vi "Convert 2D Array to Cluster.vi"(8 "error in (no error)":errorcluster, 11 "Array in":string[][](array[string])) -> (0 "error out":errorcluster, 3 "Array out":T1[](array[typedef]))   [LabVIEW 2025, in "Project.lvclass"]
doc: "Convert 2D Array of strings to Sorted, Structured Cluster of:\n\nFPGA Targets\n-Owned Modules\n--Owned Signals"
uses:
  Project.lvclass
  FPGA Settings.ctl
  Module/Module/Module Settings.ctl
  Signal/Signal/Signal Settings.ctl
  Project.lvclass/Project.ctl
  Signal/Signal/Signal.lvclass
  Module/Module/Module.lvclass
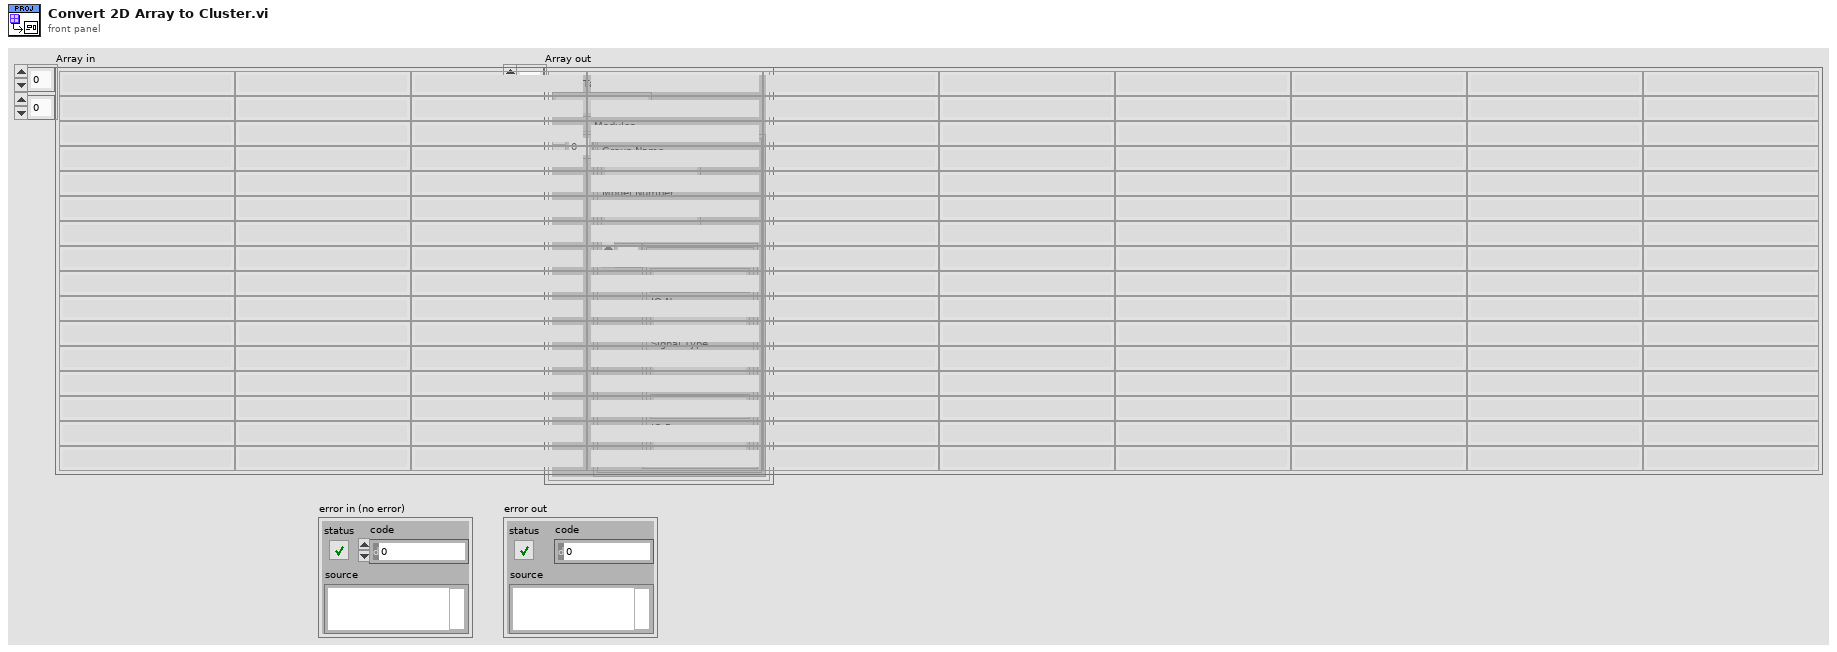
[diagram p1: front panel]
types:
  T1 = typedef "Project.lvclass/FPGA Settings.ctl" = cluster{"FPGA Target Name":string, "Modules":T2[]}
  T2 = typedef "Module.lvclass/Module Settings.ctl" = cluster{"Group Name":string, "Model Number":string, "Signals":T3[]}
  T3 = typedef "Signal.lvclass/Signal Settings.ctl" = cluster{"Signal Name":string, "IO Name":string, "Signal Type":string, "Signal Parameters":string, "IO Resource":string}
  T4 = cluster{"Group Name":string, "Model Number":string, "Signal LUT":variant}
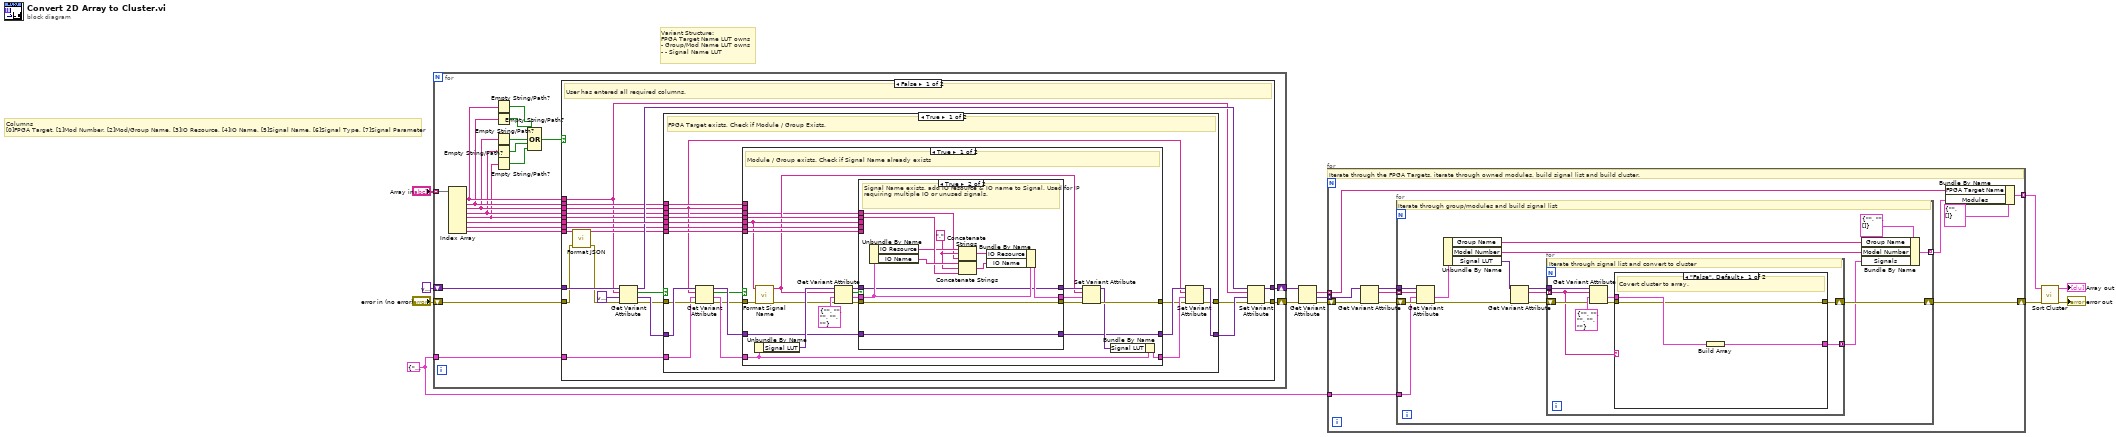
[diagram p0: block diagram]
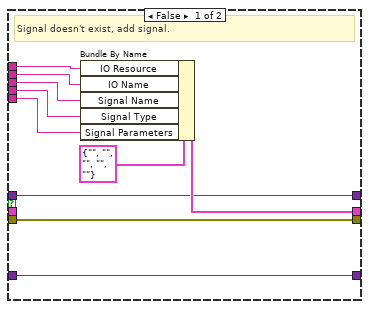
[diagram p2: hidden frame]
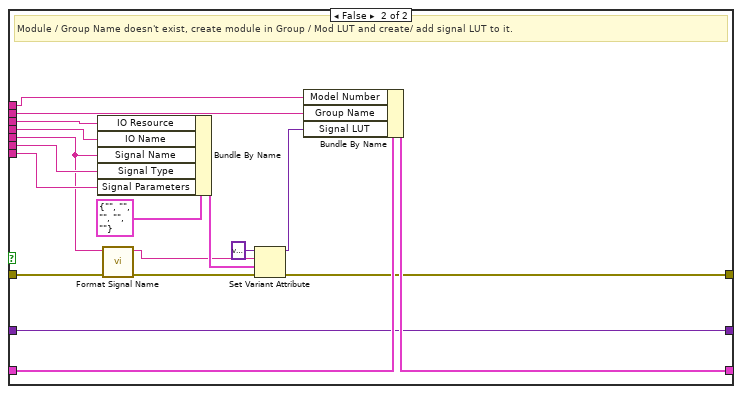
[diagram p3: hidden frame]
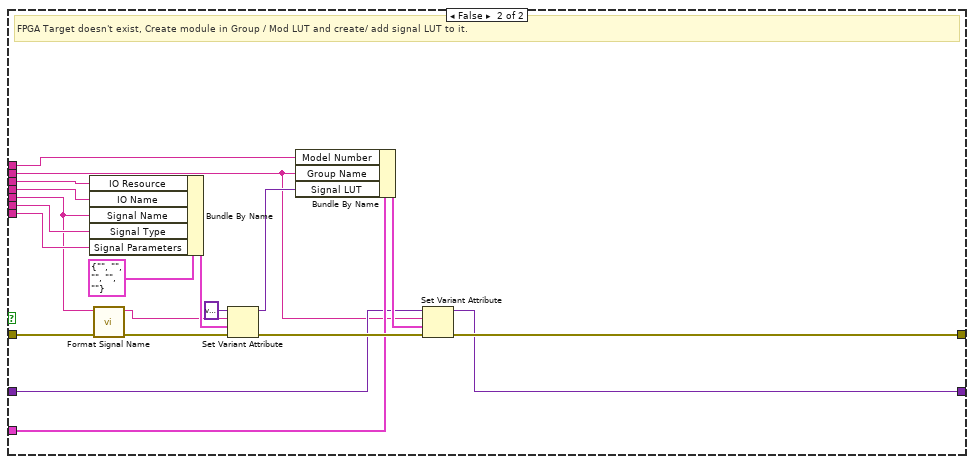
[diagram p4: hidden frame]
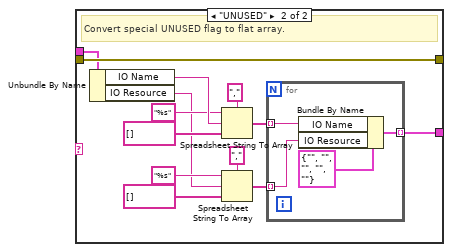
[diagram p6: hidden frame]
diagram:
  w13 = T4 {"Group Name"="", "Model Number"="", "Signal LUT"=variant}
  # "Variant Structure:\nFPGA Target Name LUT owns\n- Group/Mod Name LUT owns\n- - Signal Name LUT"
  # "Columns\n[0]FPGA Target, [1]Mod Number, [2]Mod/Group Name, [3]IO Resource, [4]IO Name, [5]Signal Name, [6]Signal Type, [7]Signal Parameter"
  n1 = for {
    tunnel: "Array in" -> [w32] mode=indexing
    shift-right: [w30] -> w8
    shift-left: variant -> [w33]
    shift-right: [w29] -> w9
    shift-left: "error in (no error)" -> [w28]
    tunnel: w13 -> [w27]
    n2 = Index Array(array=w32) -> (element #1=w24:string, element #2=w23:string, element #3=w22:string, element #4=w21:string, element #5=w20:string, element #6=w31:string, element #7=w25:string, element #8=w26:string)  [unwired: 8 in]
    n3 = Empty String/Path?(string/path=w24) -> (empty?=w19:bool)
    n4 = Empty String/Path?(string/path=w23) -> (empty?=w18:bool)
    n5 = Empty String/Path?(string/path=w22) -> (empty?=w17:bool)
    n6 = Empty String/Path?(string/path=w21) -> (empty?=w16:bool)
    n7 = Empty String/Path?(string/path=w20) -> (empty?=w15:bool)
    n8 = Compound Arithmetic op=OR(w19, w18, w17, w16, w15) -> (w14:bool)
    n9 = case shown="False" w14 {
      tunnel: w33 -> [w55 w158]
      tunnel: w31 -> [w51 _]
      tunnel: [w49 w158] -> w30
      tunnel: [w47 w159] -> w29
      tunnel: w28 -> [w43 w159]
      tunnel: w27 -> [w41 _]
      tunnel: w26 -> [w40 _]
      tunnel: w25 -> [w39 _]
      tunnel: w24 -> [w34 _]
      tunnel: w23 -> [w38 _]
      tunnel: w22 -> [w37 _]
      tunnel: w21 -> [w36 _]
      tunnel: w20 -> [w35 _]
      frame False {
        # "User has entered all required columns."
        n10 = call "Format JSON.vi"("error in (no error)"=w43, "String"=w40) -> ("error out"=w42:errorcluster, "String out"=w44:string)  [unwired: 8 in]
        n11 = Get Variant Attribute(Variant=w55, name=w34, default value (empty Variant)=variant ("default value (empty variant)"), error in=w42) -> (duplicate Variant=w45:variant, found=w54:bool, value=w52:variant, error out=w46:errorcluster)
        n12 = case shown="True" w54 {
          tunnel: w52 -> [w74 w142]
          tunnel: w36 -> [w56 w138]
          tunnel: w35 -> [w59 w147]
          tunnel: w51 -> [w60 w146]
          tunnel: w44 -> [w73 w157]
          tunnel: w37 -> [w57 w139]
          tunnel: w38 -> [w58 w140]
          tunnel: [w65 w141] -> w50
          tunnel: [w64 w155] -> w48
          tunnel: w46 -> [w63 w144]
          tunnel: w41 -> [w62 w149]
          tunnel: w39 -> [w61 w148]
          frame True {
            # "FPGA Target exists, Check if Module / Group Exists."
            n13 = Get Variant Attribute(Variant=w74, name=w57, default value (empty Variant)=w62, error in=w63) -> (duplicate Variant=w70:variant, found=w68:bool, value=w72:T4, error out=w67:errorcluster)
            n14 = case shown="True" w68 {
              tunnel: w59 -> [w97 w136]
              tunnel: w60 -> [w79 w125]
              tunnel: w61 -> [w96 w135]
              tunnel: w73 -> [w95 w134]
              tunnel: w72 -> [w83 w133]
              tunnel: [w80 w123] -> w71
              tunnel: w70 -> [w91 w123]
              tunnel: [w81 w132] -> w69
              tunnel: w67 -> [w77 w122]
              tunnel: [w85 w128] -> w66
              tunnel: w57 -> [_ w131]
              tunnel: w58 -> [_ w130]
              tunnel: w56 -> [w75 w120]
              frame True {
                # "Module / Group exists. Check if Signal Name already exists"
                n15 = Unbundle By Name(w83) -> ("Signal LUT"=w94:variant)
                n16 = call "Format Signal Name.vi"("error in (no error)"=w77, "String"=w79) -> ("error out"=w76:errorcluster, "String out"=w78:string)  [unwired: 8 in]
                n17 = Get Variant Attribute(Variant=w94, name=w78, default value (empty Variant)=T3 {"Signal Name"="", "IO Name"="", "Signal Type"="", "Signal Parameters"="", "IO Resource"=""}, error in=w76) -> (duplicate Variant=w90:variant, found=w92:bool, value=w89:T3, error out=w88:errorcluster)
                n18 = case shown="True" w92 {
                  tunnel: w97 -> [w106 w117]
                  tunnel: w96 -> [w105 _]
                  tunnel: w95 -> [w104 _]
                  tunnel: w79 -> [w103 _]
                  tunnel: w91 -> [w100 w119]
                  tunnel: w90 -> [w99 w112]
                  tunnel: w89 -> [_ w116]
                  tunnel: w88 -> [w101 w114]
                  tunnel: [w102 w113] -> w87
                  tunnel: [w101 w114] -> w86
                  tunnel: [w99 w112] -> w84
                  tunnel: [w100 w119] -> w80
                  tunnel: w75 -> [w98 w109]
                  frame False {
                    # "Signal doesn't exist, add signal."
                    n19 = Bundle By Name(cluster=T3 {"Signal Name"="", "IO Name"="", "Signal Type"="", "Signal Parameters"="", "IO Resource"=""}, "IO Resource"=w98, "IO Name"=w106, "Signal Name"=w103, "Signal Type"=w105, "Signal Parameters"=w104) -> (w102:T3)
                  }
                  frame True {
                    w110 = "," ("string")
                    # "Signal Name exists, add IO resource & IO name to Signal. Used for IP requiring multiple IO or unused signals."
                    n20 = Unbundle By Name(w116) -> ("IO Resource"=w111:string, "IO Name"=w118:string)
                    n21 = Concatenate Strings(w111, w110, w109) -> (w108:string)
                    n22 = Concatenate Strings(w118, w110, w117) -> (w115:string)
                    n23 = Bundle By Name(cluster=w116, "IO Resource"=w108, "IO Name"=w115) -> (w113:T3)
                  }
                }
                n24 = Set Variant Attribute(Variant=w84, name=w78, value=w87, error in=w86) -> (Variant out=w82:variant, error out=w85:errorcluster)  [unwired: 1 out]
                n25 = Bundle By Name(cluster=w83, "Signal LUT"=w82) -> (w81:T4)
              }
              frame False {
                # "Module / Group Name doesn't exist, create module in Group / Mod LUT and create/ add signal LUT to it."
                n26 = Bundle By Name(cluster=T3 {"Signal Name"="", "IO Name"="", "Signal Type"="", "Signal Parameters"="", "IO Resource"=""}, "IO Resource"=w120, "IO Name"=w136, "Signal Name"=w125, "Signal Type"=w135, "Signal Parameters"=w134) -> (w129:T3)
                n27 = call "Format Signal Name.vi"("error in (no error)"=w122, "String"=w125) -> ("error out"=w121:errorcluster, "String out"=w124:string)  [unwired: 8 in]
                n28 = Set Variant Attribute(Variant=variant ("variant"), name=w124, value=w129, error in=w121) -> (Variant out=w126:variant, error out=w128:errorcluster)  [unwired: 1 out]
                n29 = Bundle By Name(cluster=w133, "Model Number"=w130, "Group Name"=w131, "Signal LUT"=w126) -> (w132:T4)
              }
            }
            n30 = Set Variant Attribute(Variant=w71, name=w57, value=w69, error in=w66) -> (Variant out=w65:variant, error out=w64:errorcluster)  [unwired: 1 out]
          }
          frame False {
            # "FPGA Target doesn't exist, Create module in Group / Mod LUT and create/ add signal LUT to it."
            n31 = Bundle By Name(cluster=T3 {"Signal Name"="", "IO Name"="", "Signal Type"="", "Signal Parameters"="", "IO Resource"=""}, "IO Resource"=w138, "IO Name"=w147, "Signal Name"=w146, "Signal Type"=w148, "Signal Parameters"=w157) -> (w153:T3)
            n32 = call "Format Signal Name.vi"("error in (no error)"=w144, "String"=w146) -> ("error out"=w143:errorcluster, "String out"=w145:string)  [unwired: 8 in]
            n33 = Set Variant Attribute(Variant=variant ("variant"), name=w145, value=w153, error in=w143) -> (Variant out=w151:variant, error out=w150:errorcluster)  [unwired: 1 out]
            n34 = Bundle By Name(cluster=w149, "Model Number"=w140, "Group Name"=w139, "Signal LUT"=w151) -> (w156:T4)
            n35 = Set Variant Attribute(Variant=w142, name=w139, value=w156, error in=w150) -> (Variant out=w141:variant, error out=w155:errorcluster)  [unwired: 1 out]
          }
        }
        n36 = Set Variant Attribute(Variant=w45, name=w34, value=w50, error in=w48) -> (Variant out=w49:variant, error out=w47:errorcluster)  [unwired: 1 out]
      }
      frame True {
        # "Filter out any rows that have blanks in required columns. User isn't using."
      }
    }
  }
  n37 = Get Variant Attribute(Variant=w8, error in=w9) -> (names=w10:string[], values=w11:variant[], error out=w12:errorcluster)  [unwired: 2 in, 1 out]
  n38 = for {
    tunnel: w10 -> [w169] mode=indexing
    tunnel: w11 -> [w168] mode=indexing
    shift-right: [w164] -> w3
    shift-left: w12 -> [w167]
    tunnel: [w163] -> w4 mode=indexing
    tunnel: w13 -> [w161]
    # "Iterate through the FPGA Targets, iterate through owned modules, build signal list and build cluster."
    n39 = Get Variant Attribute(Variant=w168, error in=w167) -> (duplicate Variant=w162:variant, names=w165:string[], error out=w166:errorcluster)  [unwired: 2 in, 1 out]
    n40 = for {
      shift-right: [w173] -> w164
      shift-left: w166 -> [w186]
      tunnel: w165 -> [w185] mode=indexing
      tunnel: w162 -> [w183]
      tunnel: w161 -> [w182]
      tunnel: [w171] -> w160 mode=indexing
      # "Iterate through group/modules and build signal list"
      n41 = Get Variant Attribute(Variant=w183, name=w185, default value (empty Variant)=w182, error in=w186) -> (value=w184:T4, error out=w177:errorcluster)  [unwired: 2 out]
      n42 = Unbundle By Name(w184) -> ("Group Name"=w180:string, "Model Number"=w179:string, "Signal LUT"=w178:variant)
      n43 = Get Variant Attribute(Variant=w178, error in=w177) -> (duplicate Variant=w176:variant, names=w175:string[], error out=w174:errorcluster)  [unwired: 2 in, 1 out]
      n44 = for {
        tunnel: w176 -> [w194]
        tunnel: w175 -> [w187] mode=indexing
        shift-right: [w189] -> w173
        shift-left: w174 -> [w192]
        tunnel: [w190] -> w172 mode=concatenating
        # "Iterate through signal list and convert to cluster"
        n45 = Get Variant Attribute(Variant=w194, name=w187, default value (empty Variant)=T3 {"Signal Name"="", "IO Name"="", "Signal Type"="", "Signal Parameters"="", "IO Resource"=""}, error in=w192) -> (value=w191:T3, error out=w188:errorcluster)  [unwired: 2 out]
        n46 = case shown="\"False\", Default" w187 {
          tunnel: w191 -> [w197 w204]
          tunnel: [w196 w203] -> w190
          tunnel: [w195 w210] -> w189
          tunnel: w188 -> [w195 w210]
          frame "False", Default {
            # "Covert cluster to array."
            n47 = Build Array(w197) -> (w196:T3[])
          }
          frame "UNUSED" {
            # "Convert special UNUSED flag to flat array."
            n48 = Unbundle By Name(w204) -> ("IO Name"=w209:string, "IO Resource"=w199:string)
            n49 = Spreadsheet String To Array(delimiter (Tab)=",", format string="%s", spreadsheet string=w209, array type (2D Dbl)=string[] []) -> (array=w205:string[])
            n50 = Spreadsheet String To Array(delimiter (Tab)=",", format string="%s", spreadsheet string=w199, array type (2D Dbl)=string[] []) -> (array=w198:string[])
            n51 = for {
              tunnel: w205 -> [w213] mode=indexing
              tunnel: [w212] -> w203 mode=indexing
              tunnel: w198 -> [w211] mode=indexing
              n52 = Bundle By Name(cluster=T3 {"Signal Name"="", "IO Name"="", "Signal Type"="", "Signal Parameters"="", "IO Resource"=""}, "IO Name"=w213, "IO Resource"=w211) -> (w212:T3)
            }
          }
        }
      }
      n53 = Bundle By Name(cluster=T2 {"Group Name"="", "Model Number"="", "Signals"=[]}, "Group Name"=w180, "Model Number"=w179, "Signals"=w172) -> (w171:T2)
    }
    n54 = Bundle By Name(cluster=T1 {"FPGA Target Name"="", "Modules"=[]} ("FPGA Settings"), "FPGA Target Name"=w169, "Modules"=w160) -> (w163:T1)
  }
  n55 = call "Sort Cluster.vi"("error in (no error)"=w3, "Array in"=w4) -> ("error out"=→"error out":errorcluster, "Array out"=→"Array out":T1[])  [unwired: 8 in]
